vi "Array.vi"() -> ()   [LabVIEW 2015]
panel:
  out "min index(es)":i32
  out "min value":dbl
  out "max index(es)":i32
  out "max value":dbl
  out "second subarray":dbl[](array[numeric])
  out "first subarray":dbl[](array[numeric])
  out "index of element":i32
  out "sorted array":dbl[](array[numeric])
  out "size(s)":i32
  in  "Array 2":dbl[](array[numeric])
  in  "Array":dbl[](array[numeric])
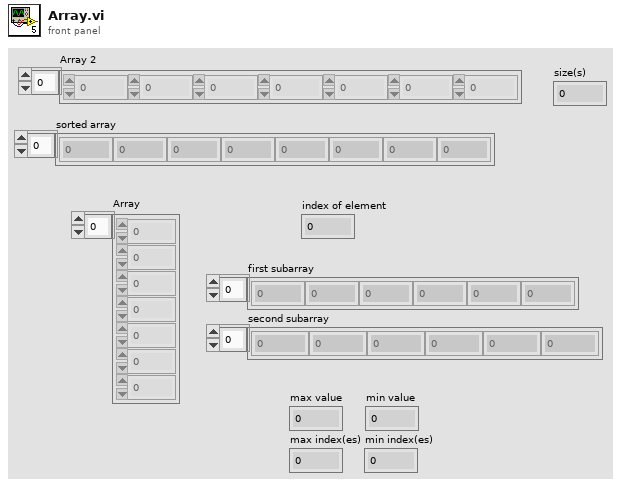
[diagram p1: front panel]
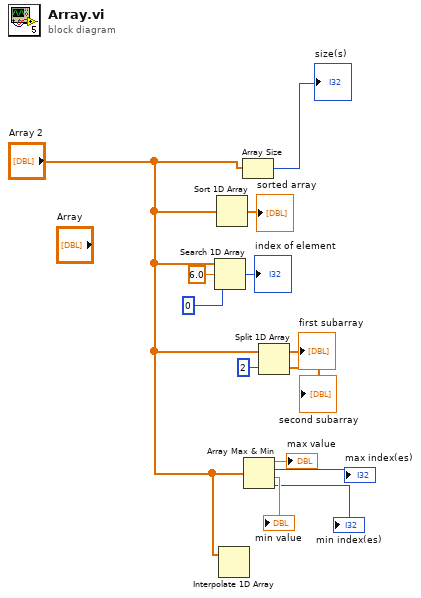
[diagram p0: block diagram]
diagram:
  n1 = Search 1D Array(1D array="Array 2", element=6.0, start index (0)=0) -> (index of element=→"index of element":i32)
  n2 = Sort 1D Array(array="Array 2") -> (sorted array=→"sorted array":dbl[])
  n3 = Interpolate 1D Array(2:"Array 2") -> ()  [unwired: 1 in, 1 out]
  n4 = Array Size(array="Array 2") -> (size(s)=→"size(s)":i32)
  n5 = Array Max & Min(array="Array 2") -> (max value=→"max value":dbl, max index (indices)=→"max index(es)":i32, min value=→"min value":dbl, min index (indices)=→"min index(es)":i32)
  n6 = Split 1D Array(array="Array 2", index=2) -> (first subarray=→"first subarray":dbl[], second subarray=→"second subarray":dbl[])
